vi "Untitled 1 (SubVI).vi"(4 "Names":T7, 5 "scopeTrace in":T8, 6 "impedance":T6, 7 "verticalrange":T2, 8 "error in (no error)":errorcluster, 9 "wfm info":T9(array[cluster]), 10 "Array":string[](array[string]), 11 "coupling":T4) -> (0 "error out":errorcluster, 3 "scopeTrace out":T8)   [LabVIEW 2011, in "PXIDigitizer.lvclass"]
uses:
  PXIDigitizer.lvclass
  ScopeTrace_String_TypDef.ctl
  impedance_Enum_TypDEf.ctl
  coupling_Enum_TypDef.ctl
  numericVariable_TypeDef.ctl
  scopeTraceInfo_TypDEf.ctl
  trace_TypDef.ctl
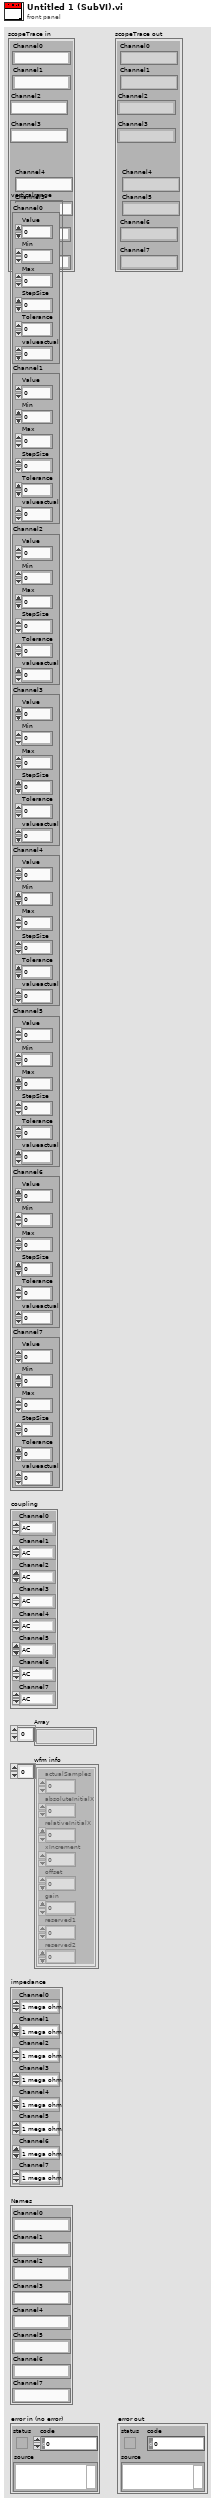
[diagram p1: front panel]
types:
  T1 = typedef "numericVariable_TypeDef.ctl" = cluster{"Value":dbl, "Min":dbl, "Max":dbl, "StepSize":dbl, "Tolerance":dbl, "valueactual":dbl}
  T2 = cluster{"Channel0":T1, "Channel1":T1, "Channel2":T1, "Channel3":T1, "Channel4":T1, "Channel5":T1, "Channel6":T1, "Channel7":T1}
  T3 = typedef "coupling_Enum_TypDef.ctl" = enum16{"AC", "DC", "Ground"}
  T4 = cluster{"Channel0":T3, "Channel1":T3, "Channel2":T3, "Channel3":T3, "Channel4":T3, "Channel5":T3, "Channel6":T3, "Channel7":T3}
  T5 = typedef "impedance_Enum_TypDEf.ctl" = enum16{"1 mega ohm", "<NA>", "50 ohms"}
  T6 = cluster{"Channel0":T5, "Channel1":T5, "Channel2":T5, "Channel3":T5, "Channel4":T5, "Channel5":T5, "Channel6":T5, "Channel7":T5}
  T7 = cluster{"Channel0":string, "Channel1":string, "Channel2":string, "Channel3":string, "Channel4":string, "Channel5":string, "Channel6":string, "Channel7":string}
  T8 = typedef "ScopeTrace_String_TypDef.ctl" = cluster{"Channel0":string, "Channel1":string, "Channel2":string, "Channel3":string, "Channel5":string, "Channel4":string, "Channel6":string, "Channel7":string}
  T9 = cluster{"actualSamples":i32, "absoluteInitialX":dbl, "relativeInitialX":dbl, "xIncrement":dbl, "offset":dbl, "gain":dbl, "reserved1":dbl, "reserved2":dbl}[]
  T10 = typedef "trace_TypDef.ctl" = cluster{"info":T11, "wfm":dbl[]}
  T11 = typedef "scopeTraceInfo_TypDEf.ctl" = cluster{"Name":string, "N":dbl, "t0":dbl, "dt":dbl, "offset":dbl, "gain":dbl, "coupling":string, "impedance":string, "range":dbl}
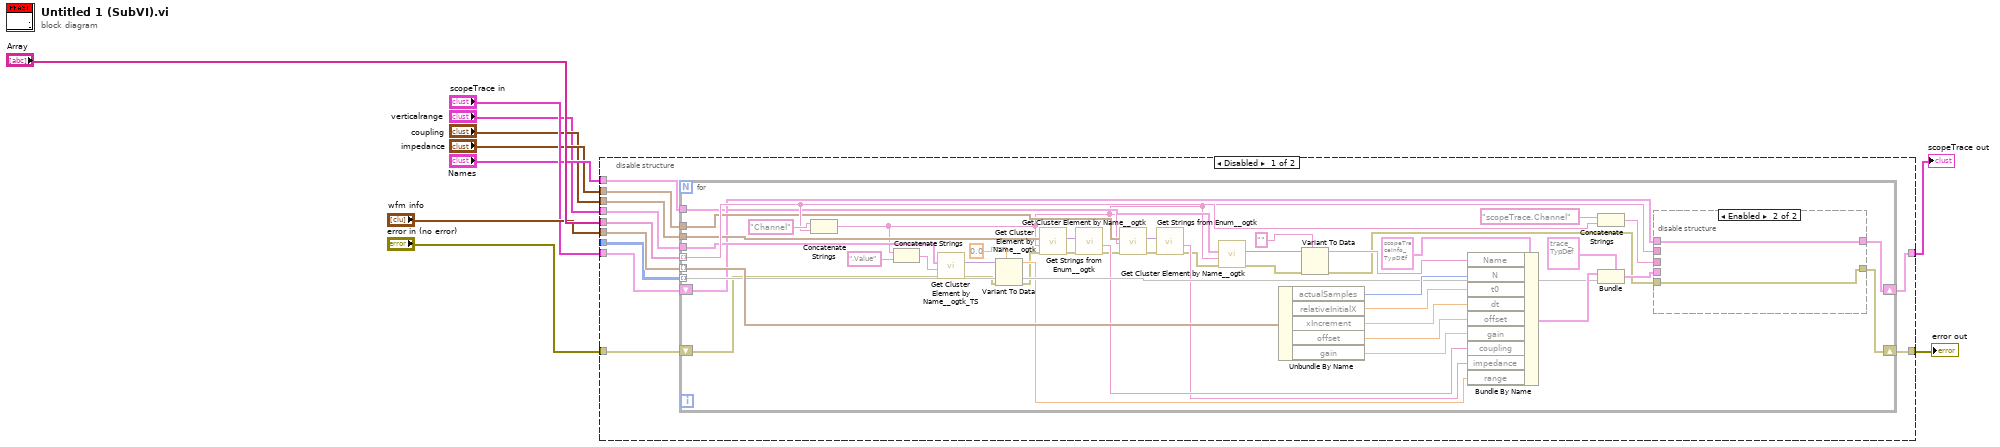
[diagram p0: block diagram]
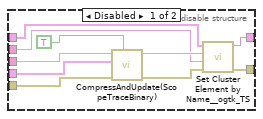
[diagram p2: hidden frame]
diagram:
  n1 = disable-structure shown="Disabled" {
    disable-tunnel: "error in (no error)" -> [w21 w78]
    disable-tunnel: "Array" -> [w20 _]
    disable-tunnel: "verticalrange" -> [w19 _]
    disable-tunnel: "coupling" -> [w18 _]
    disable-tunnel: "impedance" -> [w17 _]
    disable-tunnel: "Names" -> [w16 _]
    disable-tunnel: [w15 w79] -> w6
    disable-tunnel: "scopeTrace in" -> [w14 w79]
    disable-tunnel: [w13 w78] -> w8
    disable-tunnel: "wfm info" -> [w12 _]
    disable-tunnel: _ -> [w11 _]
    frame Disabled {
      n2 = for {
        tunnel: w12 -> [w59] mode=indexing
        tunnel: w11 -> [w58] mode=indexing
        tunnel: w20 -> [w52] mode=indexing
        shift-right: [w42] -> w13
        shift-left: w21 -> [w44]
        shift-right: [w41] -> w15
        shift-left: w14 -> [w43]
        tunnel: w19 -> [w50]
        tunnel: w18 -> [w49]
        tunnel: w17 -> [w48]
        tunnel: w16 -> [w29]
        n3 = Concatenate Strings("Channel" ("string"), w52) -> (w28:string)
        n4 = Concatenate Strings(w28, ".Value" ("string")) -> (w34:string)
        n5 = call "Get Cluster Element by Name__ogtk_TS.vi"("error in (no error)"=w44, "Element Name"=w34, "Cluster"=w50) -> ("error out"=w32:errorcluster, "VElement"=w37:variant)  [unwired: 6 in, 1 out]
        n6 = Variant To Data(error in=w32, type=0.0, Variant=w37) -> (data=w47:dbl, error out=w31:errorcluster)
        n7 = call "Get Cluster Element by Name__ogtk.vi"("error in (no error)"=w31, "Element Name"=w28, "Cluster"=w49) -> ("error out"=w39:errorcluster, "VElement"=w38:variant)  [unwired: 6 in, 1 out]
        n8 = call "Get Strings from Enum__ogtk.vi"("error in (no error)"=w39, "Enum"=w38) -> ("error out"=w30:errorcluster, "String Value"=w46:string)  [unwired: 6 in, 2 out]
        n9 = call "Get Cluster Element by Name__ogtk.vi"("error in (no error)"=w30, "Element Name"=w28, "Cluster"=w48) -> ("error out"=w33:errorcluster, "VElement"=w40:variant)  [unwired: 6 in, 1 out]
        n10 = call "Get Strings from Enum__ogtk.vi"("error in (no error)"=w33, "Enum"=w40) -> ("error out"=w26:errorcluster, "String Value"=w45:string)  [unwired: 6 in, 2 out]
        n11 = call "Get Cluster Element by Name__ogtk.vi"("error in (no error)"=w26, "Element Name"=w28, "Cluster"=w29) -> ("error out"=w27:errorcluster, "VElement"=w24:variant)  [unwired: 6 in, 1 out]
        n12 = Unbundle By Name(w59) -> ("actualSamples"=w65:i32, "relativeInitialX"=w64:dbl, "xIncrement"=w63:dbl, "offset"=w62:dbl, "gain"=w61:dbl)
        n13 = Variant To Data(error in=w27, type="", Variant=w24) -> (data=w23:string, error out=w22:errorcluster)
        n14 = Bundle By Name(cluster=T11 {"Name"="", "N"=0.0, "t0"=0.0, "dt"=0.0, "offset"=0.0, "gain"=0.0, "coupling"="", "impedance"="", "range"=0.0} ("info"), "Name"=w23, "N"=w65, "t0"=w64, "dt"=w63, "offset"=w62, "gain"=w61, "coupling"=w46, "impedance"=w45, "range"=w47) -> (w60:T11)
        n15 = Concatenate Strings("scopeTrace.Channel" ("string"), w52) -> (w51:string)
        n16 = Bundle(cluster=T10 {"info"={"Name"="", "N"=0.0, "t0"=0.0, "dt"=0.0, "offset"=0.0, "gain"=0.0, "coupling"="", "impedance"="", "range"=0.0}, "wfm"=[]} ("Scope Trace 2"), "info"=w60, "wfm"=w58) -> (w54:T10)
        n17 = disable-structure shown="Enabled" {
          disable-tunnel: w54 -> [w75 _]
          disable-tunnel: w51 -> [w74 _]
          disable-tunnel: w43 -> [w72 w77]
          disable-tunnel: [w70 w76] -> w42
          disable-tunnel: [w69 w77] -> w41
          disable-tunnel: w28 -> [w68 _]
          disable-tunnel: w22 -> [w67 w76]
          frame Disabled {
            n18 = call "CompressAndUpdate(ScopeTraceBinary).vi"("force CVT update (false)"=TRUE, "error in"=w67, "wfm"=w75, "command or variable name"=w74) -> ("error out"=w66:errorcluster, "Trace String"=w71:string)  [unwired: 6 in]
            n19 = call "Set Cluster Element by Name__ogtk_TS.vi"("error in (no error)"=w66, "Element Name (\"\": New Element Data Name)"=w68, "New Element Value"=w71, "Cluster"=w72) -> ("error out"=w70:errorcluster, "VCluster out"=w69:variant)  [unwired: 5 in, 1 out]
          }
          frame Enabled {
          }
        }
      }
    }
    frame Enabled {
    }
  }
  "error out" <- w8
  "scopeTrace out" <- w6
